vi "Parse String with TDs.vi"(8 "error in (no error)":errorcluster, 9 "offset (0)":i32, 10 "DataString":refnum<class "DataString.lvclass">, 11 "Type Descriptors":refnum<class "TD.lvclass">[](array[class])) -> (0 "error out":errorcluster, 1 "offset past parsing":i32, 2 "Array of VData":refnum<class "variant.lvclass">[](array[class]))   [LabVIEW 2020, in "variant.lvlib" / "variant.lvclass"]
doc: "Parses a flattened string with type descriptors to output an array of variant data."
uses:
  variant.lvclass
  Type Descriptor/TD.lvclass
  DataString/DataString.lvclass
  C:/projects/OpenG-Variant-Data-Library/source/library/Bytes/Bytes.lvclass
  Bytes/Bytes.lvclass/Bytes.ctl
  Bytes/Bytes.lvclass
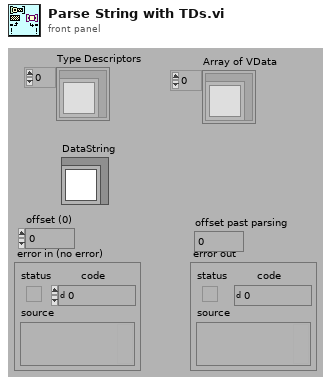
[diagram p1: front panel]
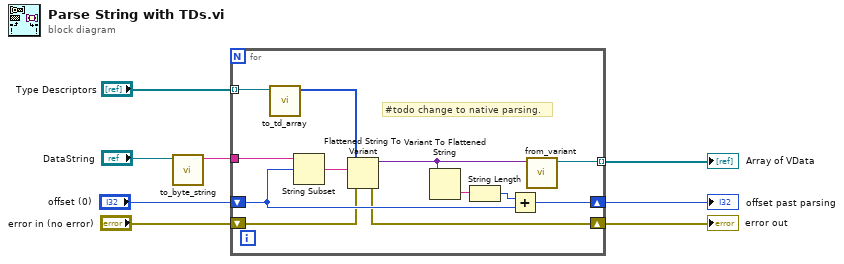
[diagram p0: block diagram]
diagram:
  n1 = call "to_byte_string.vi"("Bytes in"="DataString") -> ("byte string"=w1:string)  [unwired: 10 in]
  n2 = for {
    tunnel: w1 -> [w18]
    tunnel: [w9] -> w6 mode=indexing
    shift-right: [w15] -> w3
    shift-left: "offset (0)" -> [w17]
    shift-right: [w13] -> w5
    shift-left: "error in (no error)" -> [w14]
    tunnel: "Type Descriptors" -> [w12] mode=indexing
    # "#todo change to native parsing."
    n3 = call "to_td_array.vi"("TypeDescriptor in"=w12) -> ("type string"=w11:i16[])  [unwired: 10 in]
    n4 = String Subset(string=w18, offset (0)=w17) -> (substring=w19:string)  [unwired: 1 in]
    n5 = Flattened String To Variant(4:w14, 6:w19, 7:w11) -> (0:w13:errorcluster, 3:w10:variant)
    n6 = Variant To Flattened String(Variant=w10) -> (data string=w20:string)  [unwired: 1 out]
    n7 = String Length(string=w20) -> (length=w16:i32)
    n8 = Add(x=w16, y=w17) -> (x+y=w15:i32)
    n9 = call "from_variant.vi"("Data"=w10) -> ("LVData out"=w9:refnum<class "variant.lvclass">)  [unwired: 9 in, 1 out]
  }
  "Array of VData" <- w6
  "error out" <- w5
  "offset past parsing" <- w3
